vi "_GenerateResultTable.vi"(0 "CalResults":T1[](array[typedef])) -> (1 "ResultTable":string[][](array[string]), 2 "RefMass":dbl[](array[numeric]), 3 "MassShift":dbl[](array[numeric]), 4 "PeakWidth":dbl[](array[numeric]))   [LabVIEW 2015]
uses:
  Type/_CalibrationResult.ctl
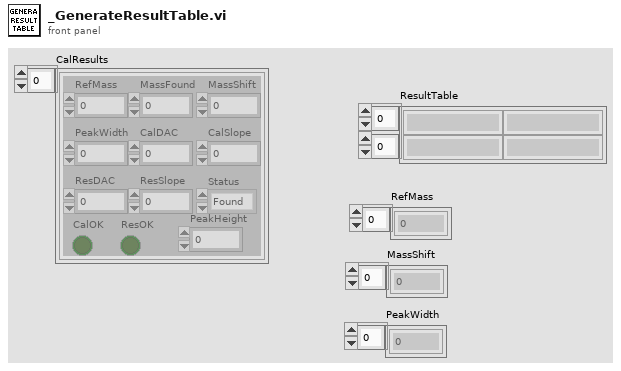
[diagram p1: front panel]
types:
  T1 = typedef "_CalibrationResult.ctl" = cluster{"RefMass":dbl, "MassFound":dbl, "MassShift":dbl, "PeakWidth":dbl, "CalDAC":dbl, "CalSlope":dbl, "ResDAC":dbl, "ResSlope":dbl, "Status":enum16{"Found", "Missing", "Not Used"}, "CalOK":bool, "ResOK":bool, "PeakHeight":dbl}
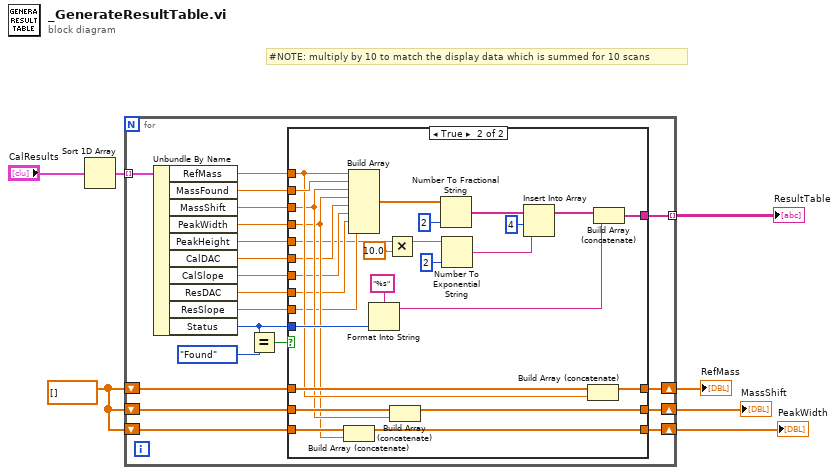
[diagram p0: block diagram]
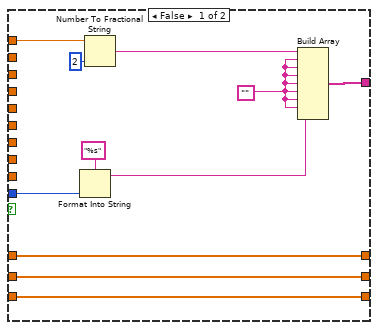
[diagram p2: hidden frame]
diagram:
  w5 = dbl[] [] ("RefMass")
  # "#NOTE: multiply by 10 to match the display data which is summed for 10 scans"
  n1 = Sort 1D Array(array="CalResults") -> (sorted array=w1:T1[])
  n2 = for {
    tunnel: w1 -> [w27] mode=indexing
    tunnel: [w19] -> w6 mode=indexing
    shift-right: [w15] -> w4
    shift-left: w5 -> [w18]
    shift-right: [w14] -> w3
    shift-left: w5 -> [w17]
    shift-right: [w13] -> w2
    shift-left: w5 -> [w16]
    n3 = Unbundle By Name(w27) -> ("RefMass"=w23:dbl, "MassFound"=w22:dbl, "MassShift"=w21:dbl, "PeakWidth"=w20:dbl, "PeakHeight"=w12:dbl, "CalDAC"=w11:dbl, "CalSlope"=w10:dbl, "ResDAC"=w9:dbl, "ResSlope"=w8:dbl, "Status"=w24:enum16{"Found", "Missing", "Not Used"})
    n4 = Equal?(x=w24, y=enum16{"Found", "Missing", "Not Used"}."Found") -> (x = y?=w25:bool)
    n5 = case shown="True" w25 {
      tunnel: w24 -> [w35 w62]
      tunnel: w23 -> [w37 w55]
      tunnel: w22 -> [_ w66]
      tunnel: w21 -> [_ w54]
      tunnel: w20 -> [_ w53]
      tunnel: w12 -> [_ w44]
      tunnel: w11 -> [_ w49]
      tunnel: w10 -> [_ w48]
      tunnel: w9 -> [_ w47]
      tunnel: [w34 w59] -> w19
      tunnel: w18 -> [w30 w58]
      tunnel: w17 -> [w29 w57]
      tunnel: w16 -> [w28 w56]
      tunnel: [w30 w52] -> w15
      tunnel: [w29 w51] -> w14
      tunnel: [w28 w50] -> w13
      tunnel: w8 -> [_ w46]
      frame False {
        w31 = ""
        n6 = Format Into String(format string="%s", w35) -> (resulting string=w32:string)  [unwired: 2 in, 1 out]
        n7 = Number To Fractional String(number=w37, precision (6)=i16 2) -> (F-format string=w33:string)  [unwired: 2 in]
        n8 = Build Array(w33, w31, w31, w31, w31, w31, w31, w31, w32) -> (w34:string[])
      }
      frame True {
        n9 = Build Array (concatenate)(w56, w53) -> (w50:dbl[])
        n10 = Build Array(w55, w66, w54, w53, w49, w48, w47, w46) -> (w65:dbl[])
        n11 = Format Into String(format string="%s", w62) -> (resulting string=w60:string)  [unwired: 2 in, 1 out]
        n12 = Multiply(x=w44, y=10.0) -> (x*y=w40:dbl)
        n13 = Build Array (concatenate)(w57, w54) -> (w51:dbl[])
        n14 = Number To Fractional String(number=w65, precision (6)=i16 2) -> (F-format string=w63:string[])  [unwired: 2 in]
        n15 = Number To Exponential String(number=w40, precision (6)=i16 2) -> (E-format string=w42:string)  [unwired: 2 in]
        n16 = Insert Into Array(array=w63, index=4, new element=w42) -> (w43:string[])
        n17 = Build Array (concatenate)(w58, w55) -> (w52:dbl[])
        n18 = Build Array (concatenate)(w43, w60) -> (w59:string[])
      }
    }
  }
  "ResultTable" <- w6
  "RefMass" <- w4
  "MassShift" <- w3
  "PeakWidth" <- w2
